vi "Format MAC ADDRESS.vi"(11 "source MAC address":cluster{u8, u8, u8, u8, u8, u8} {"?" format="%.0x"; "?" format="%.0x"; "?" format="%.0x"; "?" format="%.0x"; "?" format="%.0x"; "?" format="%.0x"}) -> (3 "spreadsheet string":string)   [LabVIEW 2025, in "Automotive Ethernet Bus Monitor UI.lvlib"]
uses:
  Automotive Ethernet Bus Monitor UI.lvlib
  <vilib>/Utility/error.llb/whitespace.ctl
  <vilib>/Utility/error.llb/Trim Whitespace One-Sided.vi
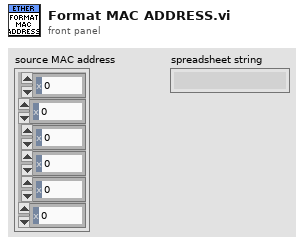
[diagram p1: front panel]
types:
  T1 = typedef "whitespace.ctl" = u16
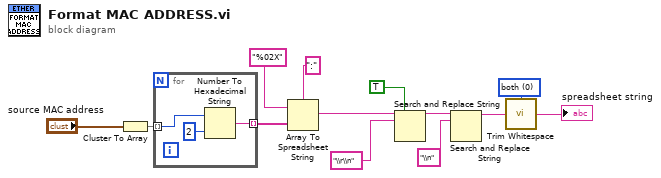
[diagram p0: block diagram]
diagram:
  w3 = T1 0 items=["both", "start of string", "end of string"] ("location (both)")
  n1 = Cluster To Array(cluster="source MAC address") -> (array=w12:u8[])
  n2 = for {
    tunnel: w12 -> [w16] mode=indexing
    tunnel: [w15] -> w9 mode=indexing
    n3 = Number To Hexadecimal String(1:i16 2 ("width (-)"), 2:w16) -> (0:w15:string)
  }
  n4 = Array To Spreadsheet String(delimiter (Tab)=":", array=w9, 3:"%02X" ("format string")) -> (spreadsheet string=w4:string)
  n5 = Search and Replace String(replace all?=TRUE ("replace all? (F)"), input string=w4, search string="\\r\\n") -> (result string=w6:string)  [unwired: 5 in, 3 out]
  n6 = Search and Replace String(input string=w6, search string="\\n") -> (result string=w2:string)  [unwired: 6 in, 3 out]
  n7 = call <vilib>:"Trim Whitespace.vi"("string"=w2, "location (both)"=w3) -> ("trimmed string"=→"spreadsheet string":string)
